vi "Read Device_Name.vi"(8 "error in (no error)":errorcluster, 11 "Processor in":refnum<class "Processor.lvclass">) -> (0 "error out":errorcluster, 2 "Device_Name":string, 3 "Processor out":refnum<class "Processor.lvclass">)   [LabVIEW 2025, in "Processor.lvclass"]
uses:
  Processor.lvclass
  Processor.lvclass/Processor.ctl
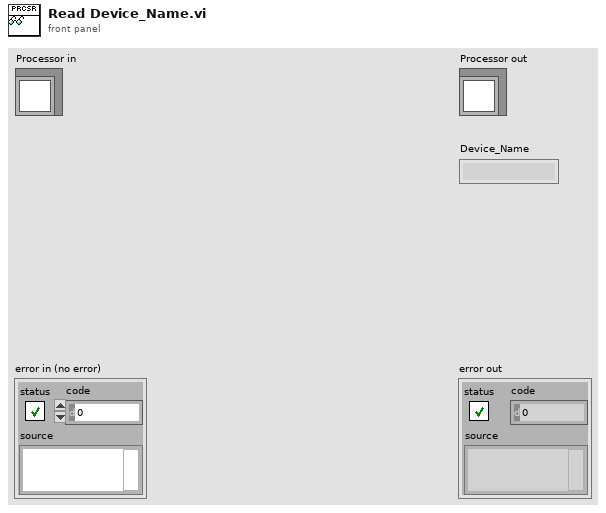
[diagram p1: front panel]
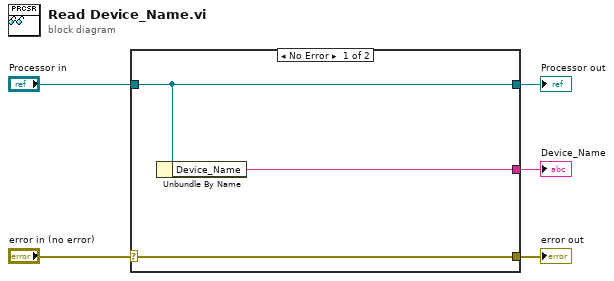
[diagram p0: block diagram]
diagram:
  n1 = case shown="No Error" "error in (no error)" {
    selector: "error in (no error)" -> [w8 w9]
    tunnel: [w8 w9] -> w4
    tunnel: [w7 w10] -> w2
    tunnel: "Processor in" -> [w7 w10]
    tunnel: [w6 _] -> w1
    frame No Error {
      n2 = Unbundle By Name(w7) -> ("Device_Name"=w6:string)
    }
    frame Error {
    }
  }
  "error out" <- w4
  "Processor out" <- w2
  "Device_Name" <- w1
